vi "Go To Destroy.vi"(7 "Sender":refnum<class "Sender.lvclass">) -> (2 "Msg":refnum<class "Msg.lvclass">)   [LabVIEW 2020, in "jettl.lvlib" / "Go To Destroy Msg.lvlib"]
uses:
  Go To Destroy Msg.lvlib
  Msg/Msg.lvclass
  Sender/Sender/Sender.lvclass
  Go To Destroy Msg/Go To Destroy Msg.lvclass
  C:/git/jettl/src/jettl/jettl/Msg/Msg.lvclass
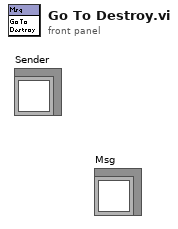
[diagram p1: front panel]
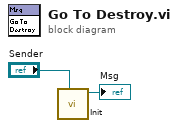
[diagram p0: block diagram]
diagram:
  n1 = call "Init.vi"("Sender"="Sender") -> ("Go To Destroy Msg out"=→"Msg":refnum<class "Go To Destroy Msg.lvclass">)  [unwired: 10 in]
